vi "create tracking boxes for image.vi"(8 "spot locations":T3[](array[typedef]), 11 "scaling info":T2={" scan settings"={"z resolution (pixels)"=0, "iterations per pixel"=0, "iterations per z-scan (=zres*iterperpixel)"=0, "x resolution (pixels)"=0, "y resolution (pixels)"=0, "number of z-lines per volume"=0, "number of repetitions (volumes)"=0, "Pockels cell voltage (bits)"=0, "Vx center (bits)"=0, "Vy center (bits)"=0, "Vx amplitude (bits)"=0, "Vy amplitude (bits)"=0, "lines to delay between scan start and output"=0, "LSB has acquire control"=FALSE}, "scale factors (um/level)"=[0.016, 0.016, 0.00025], "z-feedback range"=2560, "r sphere/sigma"=180.0}) -> (3 "Overlay Rectangles":T4(array[cluster]))   [LabVIEW 2010]
uses:
  spot location.ctl
  scan_specification_tagResonant.ctl
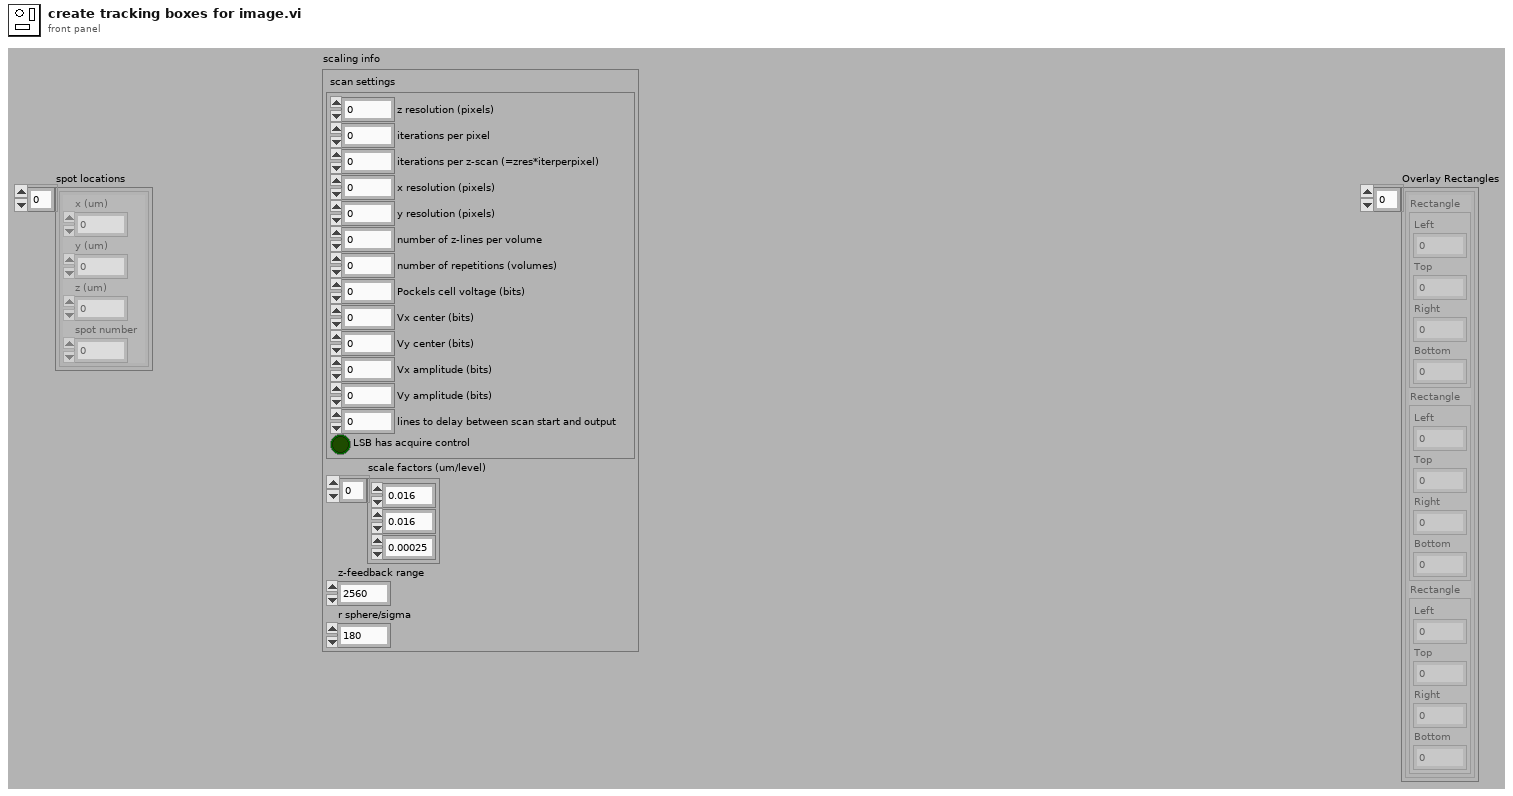
[diagram p1: front panel]
types:
  T1 = typedef "scan_specification_tagResonant.ctl" = cluster{"z resolution (pixels)":u16, "iterations per pixel":u16, "iterations per z-scan (=zres*iterperpixel)":u16, "x resolution (pixels)":u16, "y resolution (pixels)":u16, "number of z-lines per volume":u16, "number of repetitions (volumes)":i32, "Pockels cell voltage (bits)":i16, "Vx center (bits)":i16, "Vy center (bits)":i16, "Vx amplitude (bits)":i16, "Vy amplitude (bits)":i16, "lines to delay between scan start and output":u16, "LSB has acquire control":bool}
  T2 = cluster{" scan settings":T1, "scale factors (um/level)":dbl[], "z-feedback range":i16, "r sphere/sigma":dbl}
  T3 = typedef "spot location.ctl" = cluster{"x (um)":dbl, "y (um)":dbl, "z (um)":dbl, "spot number":u8}
  T4 = cluster{"Rectangle":cluster{"Left":i32, "Top":i32, "Right":i32, "Bottom":i32}, "Rectangle":cluster{"Left":i32, "Top":i32, "Right":i32, "Bottom":i32}, "Rectangle":cluster{"Left":i32, "Top":i32, "Right":i32, "Bottom":i32}}[]
  T5 = cluster{"Left":i32, "Top":i32, "Right":i32, "Bottom":i32}
  T6 = cluster{"Rectangle":cluster{"Left":i32, "Top":i32, "Right":i32, "Bottom":i32}, "Rectangle":cluster{"Left":i32, "Top":i32, "Right":i32, "Bottom":i32}, "Rectangle":cluster{"Left":i32, "Top":i32, "Right":i32, "Bottom":i32}}
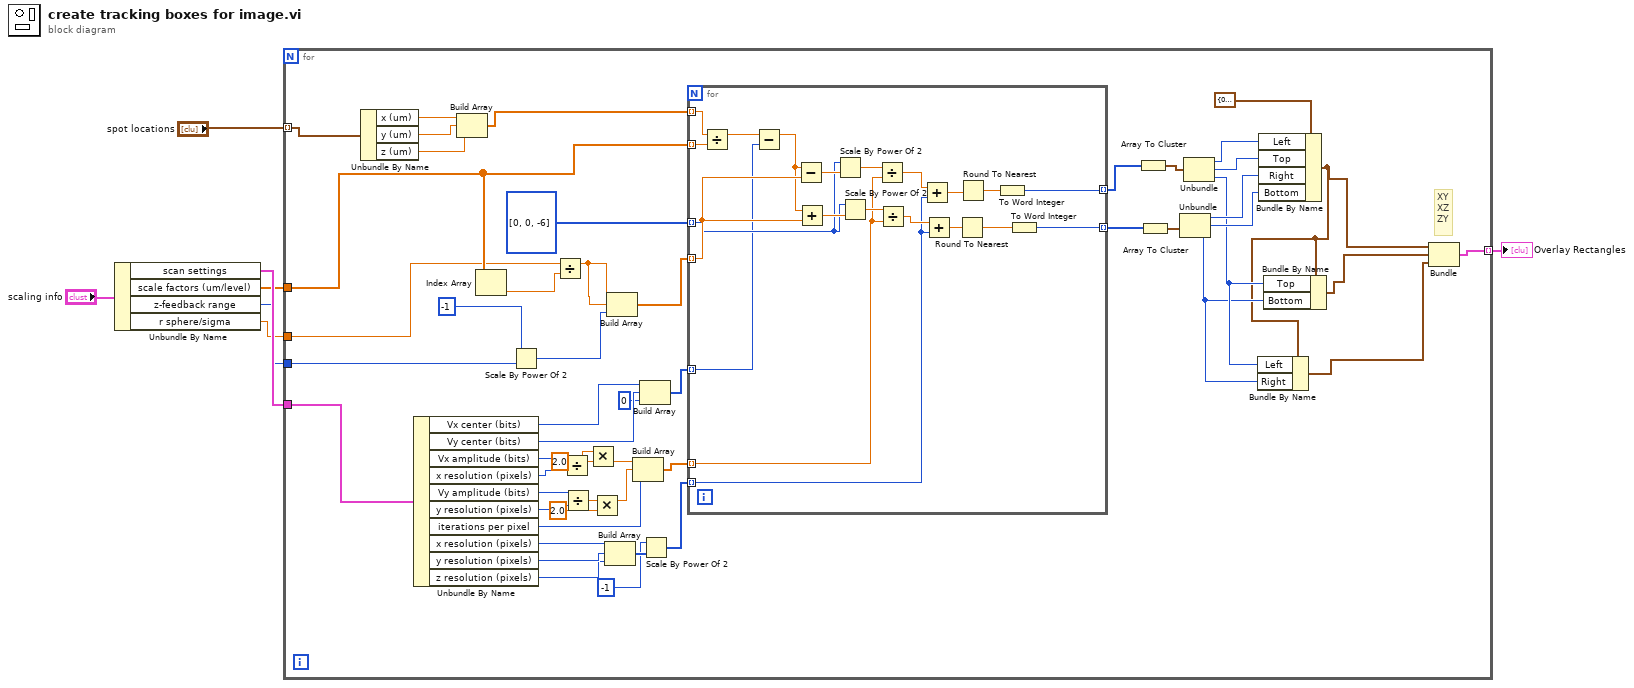
[diagram p0: block diagram]
diagram:
  n1 = Unbundle By Name("scaling info") -> ("scan settings"=w4:T1, "scale factors (um/level)"=w3:dbl[], "z-feedback range"=w2:i16, "r sphere/sigma"=w1:dbl)
  n2 = for {
    tunnel: [w24] -> w7 mode=indexing
    tunnel: "spot locations" -> [w18] mode=indexing
    tunnel: w4 -> [w11]
    tunnel: w3 -> [w10]
    tunnel: w2 -> [w9]
    tunnel: w1 -> [w8]
    # "XY\nXZ\nZY"
    n3 = Unbundle By Name(w18) -> ("x (um)"=w17:dbl, "y (um)"=w16:dbl, "z (um)"=w15:dbl)
    n4 = Unbundle By Name(w11) -> ("Vx center (bits)"=w57:i16, "Vy center (bits)"=w56:i16, "Vx amplitude (bits)"=w50:i16, "x resolution (pixels)"=w51:u16, "Vy amplitude (bits)"=w49:i16, "y resolution (pixels)"=w48:u16, "iterations per pixel"=w46:u16, "x resolution (pixels)"=w44:u16, "y resolution (pixels)"=w43:u16, "z resolution (pixels)"=w42:u16)
    n5 = Build Array(w17, w16, w15) -> (w14:dbl[])
    n6 = Index Array(array=w10) -> (element=w12:dbl)  [unwired: 1 in]
    n7 = Scale By Power Of 2(n=-1, x=w9) -> (x*2^n=w53:i16)
    n8 = Divide(x=w8, y=w12) -> (x/y=w13:dbl)
    n9 = Divide(x=w50, y=w51) -> (x/y=w22:dbl)
    n10 = Divide(x=w49, y=w48) -> (x/y=w47:dbl)
    n11 = Multiply(x=w22, y=2.0) -> (x*y=w23:dbl)
    n12 = Multiply(x=w47, y=2.0) -> (x*y=w20:dbl)
    n13 = Build Array(w44, w43, w42) -> (w41:u16[])
    n14 = Build Array(w13, w13, w53) -> (w58:dbl[])
    n15 = Build Array(w23, w20, w46) -> (w45:dbl[])
    n16 = Build Array(w57, w56, i16 0 ("element")) -> (w54:i16[])
    n17 = Scale By Power Of 2(n=-1, x=w41) -> (x*2^n=w39:u16[])
    n18 = for {
      tunnel: i32[] [0, 0, -6] -> [w77] mode=indexing
      tunnel: w14 -> [w62] mode=indexing
      tunnel: w58 -> [w80] mode=indexing
      tunnel: w54 -> [w75] mode=indexing
      tunnel: w45 -> [w72] mode=indexing
      tunnel: w39 -> [w69] mode=indexing
      tunnel: [w64] -> w38 mode=indexing
      tunnel: [w63] -> w37 mode=indexing
      tunnel: w10 -> [w60] mode=indexing
      n19 = Divide(x=w62, y=w60) -> (x/y=w61:dbl)
      n20 = Subtract(x=w61, y=w75) -> (x-y=w76:dbl)
      n21 = Subtract(x=w76, y=w80) -> (x-y=w79:dbl)
      n22 = Add(x=w76, y=w80) -> (x+y=w78:dbl)
      n23 = Scale By Power Of 2(n=w77, x=w79) -> (x*2^n=w74:dbl)
      n24 = Scale By Power Of 2(n=w77, x=w78) -> (x*2^n=w73:dbl)
      n25 = Divide(x=w74, y=w72) -> (x/y=w71:dbl)
      n26 = Divide(x=w73, y=w72) -> (x/y=w70:dbl)
      n27 = Add(x=w71, y=w69) -> (x+y=w68:dbl)
      n28 = Add(x=w70, y=w69) -> (x+y=w67:dbl)
      n29 = Round To Nearest(number=w67) -> (nearest integer value=w65:dbl)
      n30 = Round To Nearest(number=w68) -> (nearest integer value=w66:dbl)
      n31 = To Word Integer(number=w66) -> (16bit integer=w64:i16)
      n32 = To Word Integer(number=w65) -> (16bit integer=w63:i16)
    }
    n33 = Array To Cluster(array=w38) -> (cluster=w36:cluster{"[0]":i16, "[1]":i16, "[2]":i16})
    n34 = Array To Cluster(array=w37) -> (cluster=w35:cluster{"[0]":i16, "[1]":i16, "[2]":i16})
    n35 = Unbundle(w35) -> ("[0]"=w30:i16, "[1]"=w32:i16, "[2]"=w28:i16)
    n36 = Unbundle(w36) -> ("[0]"=w31:i16, "[1]"=w33:i16, "[2]"=w29:i16)
    n37 = Bundle By Name(cluster=T5 {"Left"=0, "Top"=0, "Right"=0, "Bottom"=0} ("Rectangle"), "Left"=w31, "Top"=w33, "Right"=w30, "Bottom"=w32) -> (w27:T5)
    n38 = Bundle By Name(cluster=w27, "Left"=w29, "Right"=w28) -> (w25:T5)
    n39 = Bundle By Name(cluster=w27, "Top"=w29, "Bottom"=w28) -> (w26:T5)
    n40 = Bundle("Rectangle"=w27, "Rectangle"=w26, "Rectangle"=w25) -> (w24:T6)  [unwired: 1 in]
  }
  "Overlay Rectangles" <- w7
